vi "test_libssh2_channel_set_blocking.vi"() -> ()   [LabVIEW 2013, in "libssh2_integration_tests.lvlib"]
uses:
  libssh2_integration_tests.lvlib
  <vilib>/addons/_JKI Toolkits/Caraya/classes/Test/Test.lvclass
  libssh2/libssh2.lvlib
  <vilib>/addons/_JKI Toolkits/Caraya/classes/Assert/Assert.lvclass
panel:
  out "error out":errorcluster
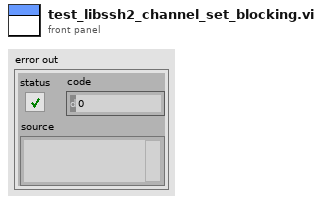
[diagram p1: front panel]
types:
  T1 = typedef "libssh2.lvlib/Session Refnum.ctl" = refnum<k1>
  T2 = typedef "libssh2.lvlib/Channel Refnum.ctl" = refnum<k1>
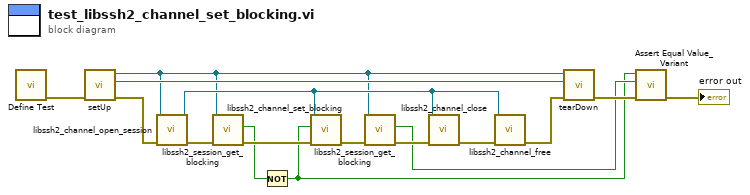
[diagram p0: block diagram]
diagram:
  n1 = call <vilib>:"Define Test.vi"() -> ("error out"=w15:errorcluster)  [unwired: 10 in, 1 out]
  n2 = call "setUp.vi"("error in (no error)"=w15) -> ("error out"=w10:errorcluster, "connection ID"=w13:refnum<k5>, "session"=w1:T1)  [unwired: 8 in]
  n3 = call "libssh2_channel_open_session.vi"("error in (no error)"=w10, "session"=w1) -> ("error out"=w7:errorcluster, "channel"=w11:T2)  [unwired: 8 in]
  n4 = call "libssh2_session_get_blocking.vi"("error in (no error)"=w7, "session"=w1) -> ("error out"=w5:errorcluster, "blocking"=w4:bool)  [unwired: 8 in]
  n5 = Not(x=w4) -> (.not. x?=w2:bool)
  n6 = call "libssh2_channel_set_blocking.vi"("error in (no error)"=w5, "blocking"=w2, "channel"=w11) -> ("error out"=w8:errorcluster)  [unwired: 8 in]
  n7 = call "libssh2_session_get_blocking.vi"("error in (no error)"=w8, "session"=w1) -> ("error out"=w6:errorcluster, "blocking"=w3:bool)  [unwired: 8 in]
  n8 = call "libssh2_channel_close.vi"("error in (no error)"=w6, "channel"=w11) -> ("error out"=w12:errorcluster)  [unwired: 9 in]
  n9 = call "libssh2_channel_free.vi"("error in (no error)"=w12, "channel"=w11) -> ("error out"=w9:errorcluster)  [unwired: 9 in]
  n10 = call "tearDown.vi"("error in (no error)"=w9, "connection ID"=w13, "session"=w1) -> ("error out"=w14:errorcluster)  [unwired: 8 in]
  n11 = call <vilib>:"Assert Equal Value_Variant.vi"("error in (no error)"=w14, "Y"=w3, "X"=w2) -> ("error out"=→"error out":errorcluster)  [unwired: 7 in, 1 out]
